vi "MNK_FP_to_DSC.vi"(8 "error in (no error)":errorcluster, 10 "str":string[](array[string]), 11 "dbl":dbl[](array[numeric])) -> (0 "error out":errorcluster)   [LabVIEW 2016]
panel:
  in  "str var":refnum<k21>[](array[refnum])=["ni.var.psp://housesoftheholy/MNK_18T/MNK_FP_STATE"]
  in  "dbl var":refnum<k21>[](array[refnum])=["ni.var.psp://housesoftheholy/MNK_18T/MNK_FP_P1", "ni.var.psp://housesoftheholy/MNK_18T/MNK_FP_P2", "ni.var.psp://housesoftheholy/MNK_18T/MNK_FP_P3", "ni.var.psp://housesoftheholy/MNK_18T/MNK_FP_P4", "ni.var.psp://housesoftheholy/MNK_18T/MNK_FP_P5", "ni.var.psp://housesoftheholy/MNK_18T/MNK_FP_P6", "ni.var.psp://housesoftheholy/MNK_18T/MNK_FP_P7", "ni.var.psp://housesoftheholy/MNK_18T/MNK_FP_Flow", "ni.var.psp://housesoftheholy/MNK_18T/MNK_FP_MG0", "ni.var.psp://housesoftheholy/MNK_18T/MNK_FP_MG1", "ni.var.psp://housesoftheholy/MNK_18T/MNK_FP_MG2", "ni.var.psp://housesoftheholy/MNK_18T/MNK_FP_MG3", "ni.var.psp://housesoftheholy/MNK_18T/MNK_FP_MG4", "ni.var.psp://housesoftheholy/MNK_18T/MNK_FP_MG5", "ni.var.psp://housesoftheholy/MNK_18T/MNK_FP_state0", "ni.var.psp://housesoftheholy/MNK_18T/MNK_FP_state1", "ni.var.psp://housesoftheholy/MNK_18T/MNK_FP_state2"]
  # "MNK FP to DSC"
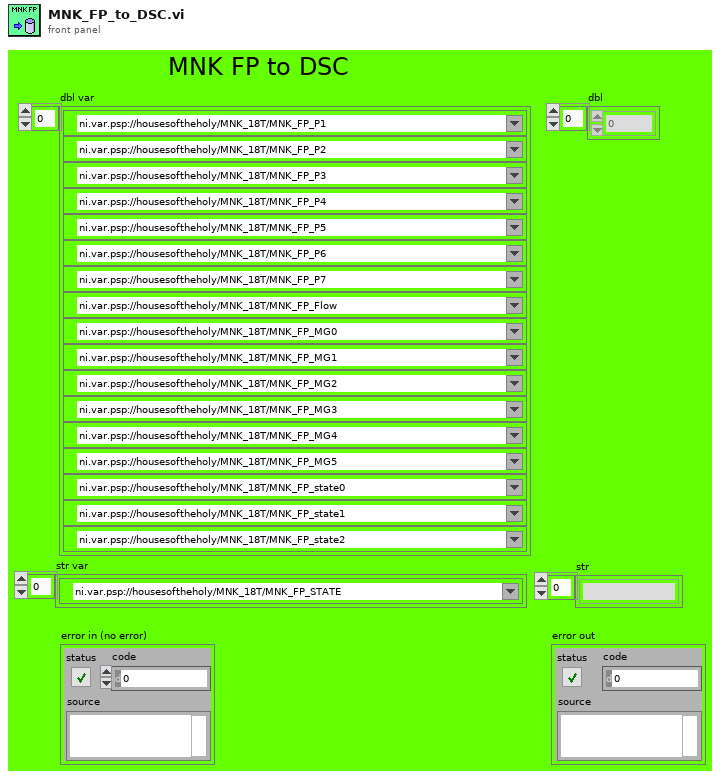
[diagram p1: front panel]
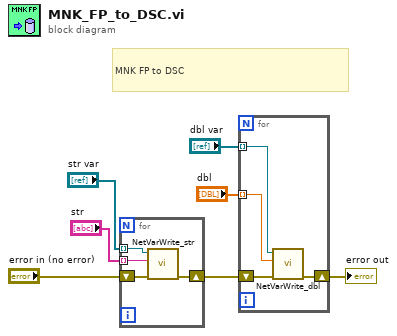
[diagram p0: block diagram]
diagram:
  # "MNK FP to DSC"
  n1 = for {
    tunnel: "str var" -> [w11] mode=indexing
    tunnel: "str" -> [w10] mode=indexing
    shift-right: [w8] -> w1
    shift-left: "error in (no error)" -> [w9]
    n2 = call "NetVarWrite_str.vi"("error in (no error)"=w9, "String"=w10, "Refnum in"=w11) -> ("error out"=w8:errorcluster)  [unwired: 8 in]
  }
  n3 = for {
    tunnel: "dbl var" -> [w14] mode=indexing
    tunnel: "dbl" -> [w15] mode=indexing
    shift-right: [w12] -> w2
    shift-left: w1 -> [w13]
    n4 = call "NetVarWrite_dbl.vi"("error in (no error)"=w13, "Numeric"=w15, "Refnum in"=w14) -> ("error out"=w12:errorcluster)  [unwired: 8 in]
  }
  "error out" <- w2
